vi "Shutter.vi"(0 "KCube Shutter Device Reference 2":refnum<vi>, 1 "Shutter Ctrls 2":refnum<vi>) -> ()   [LabVIEW 2019]
uses:
  D:/Users/manip-thz/Documents/Controle_Manip_2020/Thorlabs.MotionControl.KCube.SolenoidCLI.dll
  Thorlabs.MotionControl.KCube.SolenoidCLI.dll
panel:
  in  "KCube Shutter Device Reference":refnum<k24>
  in  "Shutter Ctrls":u16(ring)
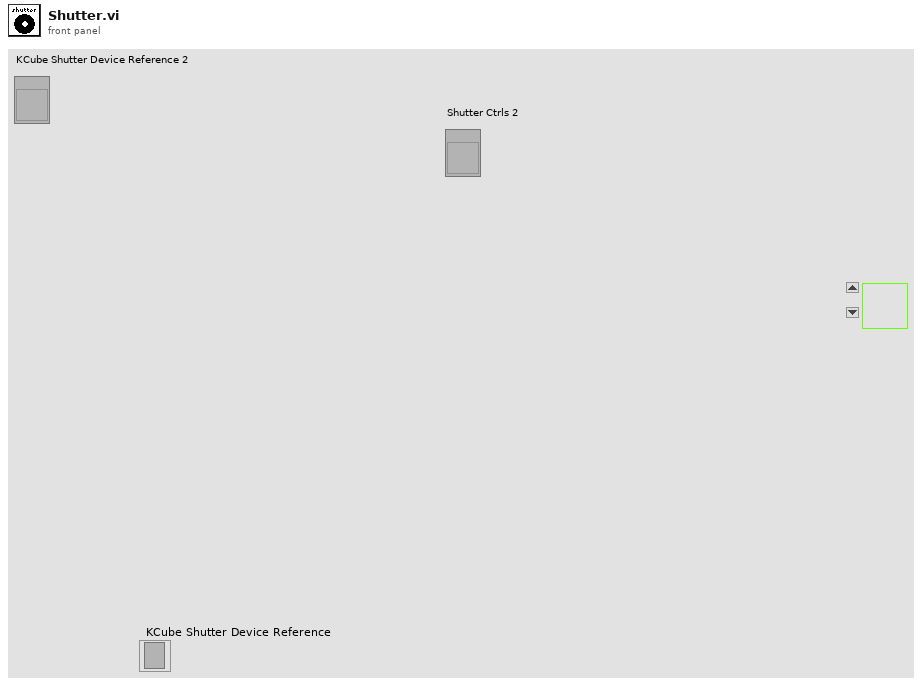
[diagram p1: front panel]
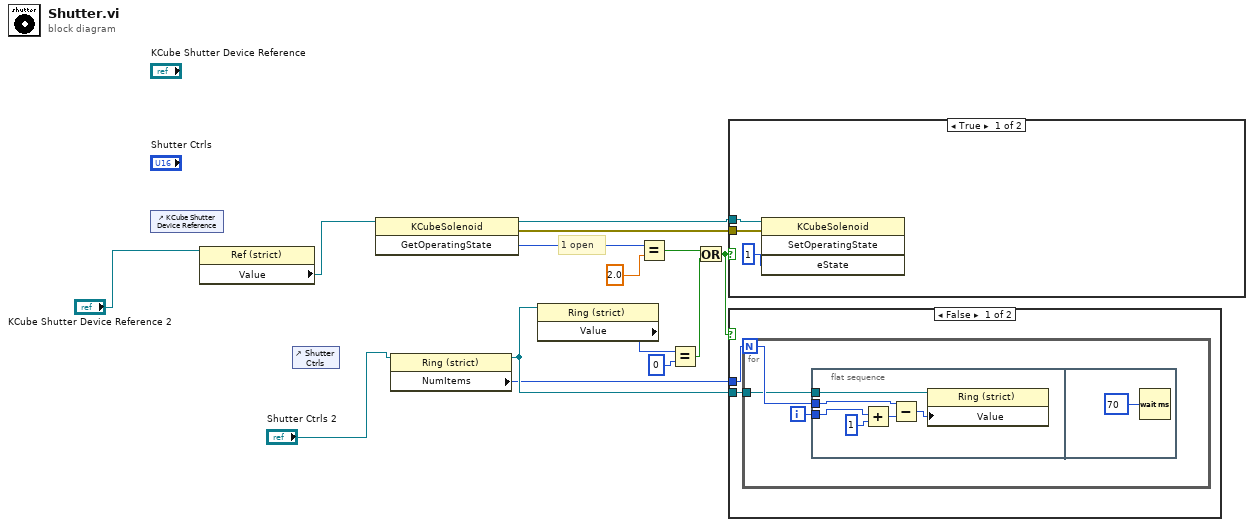
[diagram p0: block diagram]
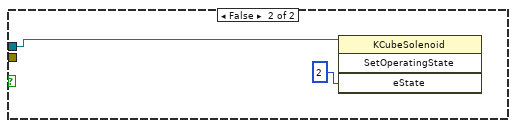
[diagram p2: hidden frame]
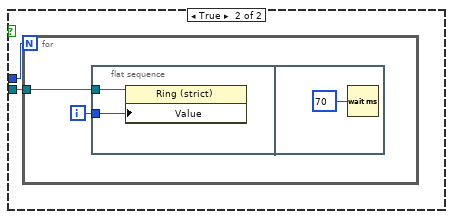
[diagram p3: hidden frame]
diagram:
  # "1 open"
  n1 = control-ref of="KCube Shutter Device Reference"() -> ()  [unwired: 1 out]
  n2 = property class="Ref (strict)"(reference="KCube Shutter Device Reference 2") -> ("Value"=w3:refnum<k24>)  [unwired: 1 in, 2 out]
  n3 = control-ref of="Shutter Ctrls"() -> ()  [unwired: 1 out]
  n4 = invoke class="KCubeSolenoid" method="GetOperatingState"(reference=w3) -> (reference out=w13:refnum<k24>, error out=w14:errorcluster, "GetOperatingState"=w12:i32)  [unwired: 2 in]
  n5 = property on="Property Node" class="Ring (strict)"(reference="Shutter Ctrls 2") -> (reference out=w5:refnum<vi>, "NumItems"=w4:u32)  [unwired: 1 in, 1 out]
  n6 = property on="Property Node" class="Ring (strict)"(reference=w5) -> ("Value"=w6:u16)  [unwired: 1 in, 2 out]
  n7 = Equal?(x=w12, y=2.0) -> (x = y?=w8:bool)
  n8 = Equal?(x=w6, y=u16 0) -> (x = y?=w9:bool)
  n9 = Or(x=w8, y=w9) -> (x .or. y?=w10:bool)
  n10 = case shown="True" w10 {
    tunnel: w13 -> [w16 w18]
    tunnel: w14 -> [w15 _]
    frame True {
      n11 = invoke class="KCubeSolenoid" method="SetOperatingState"(reference=w16, error in=w15, "eState"=1) -> ()  [unwired: 1 in, 4 out]
    }
    frame False {
      n12 = invoke class="KCubeSolenoid" method="SetOperatingState"(reference=w18, "eState"=2) -> ()  [unwired: 2 in, 4 out]
    }
  }
  n13 = case shown="False" w10 {
    tunnel: w4 -> [w20 w33]
    tunnel: w5 -> [w21 w32]
    frame False {
      n14 = for {
        N: w20 -> [w24]
        tunnel: w21 -> [w22]
        i -> [w23]
        n15 = flat-sequence {
          tunnel: w23 -> [w27]
          tunnel: w24 -> [w30]
          tunnel: w22 -> [w25]
          frame #0 {
            n16 = Add(x=w27, y=1) -> (x+y=w28:i32)
            n17 = Subtract(x=w30, y=w28) -> (x-y=w29:i32)
            n18 = property on="Property Node" class="Ring (strict)"(reference=w25, "Value"=w29) -> ()  [unwired: 1 in, 2 out]
          }
          frame #1 {
            n19 = Wait (ms)(milliseconds to wait=u32 70) -> ()  [unwired: 1 out]
          }
        }
      }
    }
    frame True {
      n20 = for {
        N: w33 -> [_]
        tunnel: w32 -> [w34]
        i -> [w35]
        n21 = flat-sequence {
          tunnel: w35 -> [w36]
          tunnel: w34 -> [w37]
          frame #0 {
            n22 = property on="Property Node" class="Ring (strict)"(reference=w37, "Value"=w36) -> ()  [unwired: 1 in, 2 out]
          }
          frame #1 {
            n23 = Wait (ms)(milliseconds to wait=u32 70) -> ()  [unwired: 1 out]
          }
        }
      }
    }
  }
